vi "BarPlot.vi"(3 "Zen Analytics in":refnum<class "Zen Analytics.lvclass">, 5 "MeasuremetDisabledIndex":i32[](array[numeric]), 6 "InitializationValue-Input":T2, 7 "Plot Cluster":T1, 8 "error in (no error)":errorcluster, 9 "Graph Refference's":T3, 10 "MeasurementInitializationData.Measurement Names":string[](array[string]), 11 "Input_Data":dbl[][](array[numeric])=[[1.0, 2.0, 3.0, 4.0, 5.0, 6.0, 7.0, 8.0, 9.0, 10.0], [1.0, 2.0, 3.0, 4.0, 5.0, 6.0, 7.0, 8.0, 9.0, 10.0], [1.0, 2.0, 3.0, 4.0, 5.0, 6.0, 7.0, 8.0, 9.0, 10.0], [1.0, 2.0, 3.0, 4.0, 5.0, 6.0, 7.0, 8.0, 9.0, 10.0], [1.0, 2.0, 3.0, 4.0, 5.0, 6.0, 7.0, 8.0, 9.0, 10.0], [1.0, 2.0, 3.0, 4.0, 5.0, 6.0, 7.0, 8.0, 9.0, 10.0], [1.0, 2.0, 3.0, 4.0, 5.0, 6.0, 7.0, 8.0, 9.0, 10.0], [1.0, 2.0, 3.0, 4.0, 5.0, 6.0, 7.0, 8.0, 9.0, 10.0], [1.0, 2.0, 3.0, 4.0, 6.0, 6.0, 7.0, 8.0, 9.0, 10.0], [1.0, 2.0, 3.0, 4.0, 5.0, 6.0, 7.0, 8.0, 9.0, 10.0]]) -> (0 "error out":errorcluster, 4 "InitializationValues-Output":T2)   [LabVIEW 2019, in "Zen Analytics.lvlib" / "Zen Analytics.lvclass"]
uses:
  Zen Analytics.lvclass
  Dependency/Plot Cluster.ctl
  Dependency/GraphReff.ctl
panel:
  in  "ColorForProduction":u32[](array[colorbox])=[30476, 12845604]
  in  "ColorsForDefects":u32[](array[colorbox])=[10387, 14090395, 38587, 9764938, 14009600, 8908544, 16618491, 12294549, 16752640, 3516387, 14559999, 10192043, 7115400, 10130292, 9071204, 9961652, 2293830, 9806267, 9069692, 10138508, 9217715, 10788291, 12293525, 16512, 8388736, 8421568, 4194432, 16384, 16448, 4194304, 8405056, 5177423, 2293830]
types:
  T1 = typedef "Zen Analytics.lvlib/Zen Analytics.lvclass/Plot Cluster.ctl" = cluster{"Reduced 2D":dbl[][], "Start Index":i32, "No Of New Termnals":i32, "Top/Bottom":bool, "Values Inserted":i32, "Re-Initialised":bool, "Statistical params":string[][], "MeasurementInitializationData":cluster{"Measurement-ID":i32[], "Measurement Names":string[], "NominalValues":dbl[], "LSL":dbl[], "USL":dbl[], "LCL":dbl[], "UCL":dbl[]}, "MeasurementData":cluster{"Measurement ID":i32, "Measurement Name":string, "Nominal Values":dbl, "LSL":dbl, "USL":dbl, "LCL":dbl, "UCL":dbl}[], "ResultData2D":dbl[][], "PlotParameters":cluster{"Trend":cluster{"TrendPlotID":dbl, "PlotProperties":cluster{"FontName":string, "FontSize":dbl, "FontColor":string, "IsBold":bool, "IsItalic":bool, "PlotColor":string}}[], "Histogram":cluster{"HistogramPlotID":dbl, "PlotProperties":cluster{"FontName":string, "FontSize":dbl, "FontColor":string, "IsBold":bool, "IsItalic":bool, "PlotColor":string}}[], "BarPlot":cluster{"BarPlotID":dbl, "BarValuesID":dbl, "PlotProperties":cluster{"FontName":string, "FontSize":dbl, "IsBold":bool, "IsItalic":bool, "FontColor":string}, "Sectors":string[]}[], "PieChart":cluster{"PieChartID":dbl, "PieChartValueID":dbl, "PlotProperties":cluster{"FontName":string, "FontSize":dbl, "IsBold":bool, "IsItalic":bool, "FontColor":string}, "Sectors":string[]}[]}}
  T2 = cluster{"InitializationDefect":dbl[], "InitializationProduction":dbl[]}
  T3 = typedef "Zen Analytics.lvlib/Zen Analytics.lvclass/GraphReff.ctl" = cluster{"HistgramGraph-reff":refnum<vi>[], "BarGraph-reff":refnum<vi>[], "PieGraph-reff":refnum<vi>[], "Lable-reff":refnum<vi>[], "TrendGraph-reff":refnum<vi>[], "CpCpkTable":refnum<vi>}
  T4 = cluster{"Measurement-ID":i32[], "Measurement Names":string[], "NominalValues":dbl[], "LSL":dbl[], "USL":dbl[], "LCL":dbl[], "UCL":dbl[]}
  T5 = cluster{"BarPlotID":dbl, "BarValuesID":dbl, "PlotProperties":cluster{"FontName":string, "FontSize":dbl, "IsBold":bool, "IsItalic":bool, "FontColor":string}, "Sectors":string[]}[]
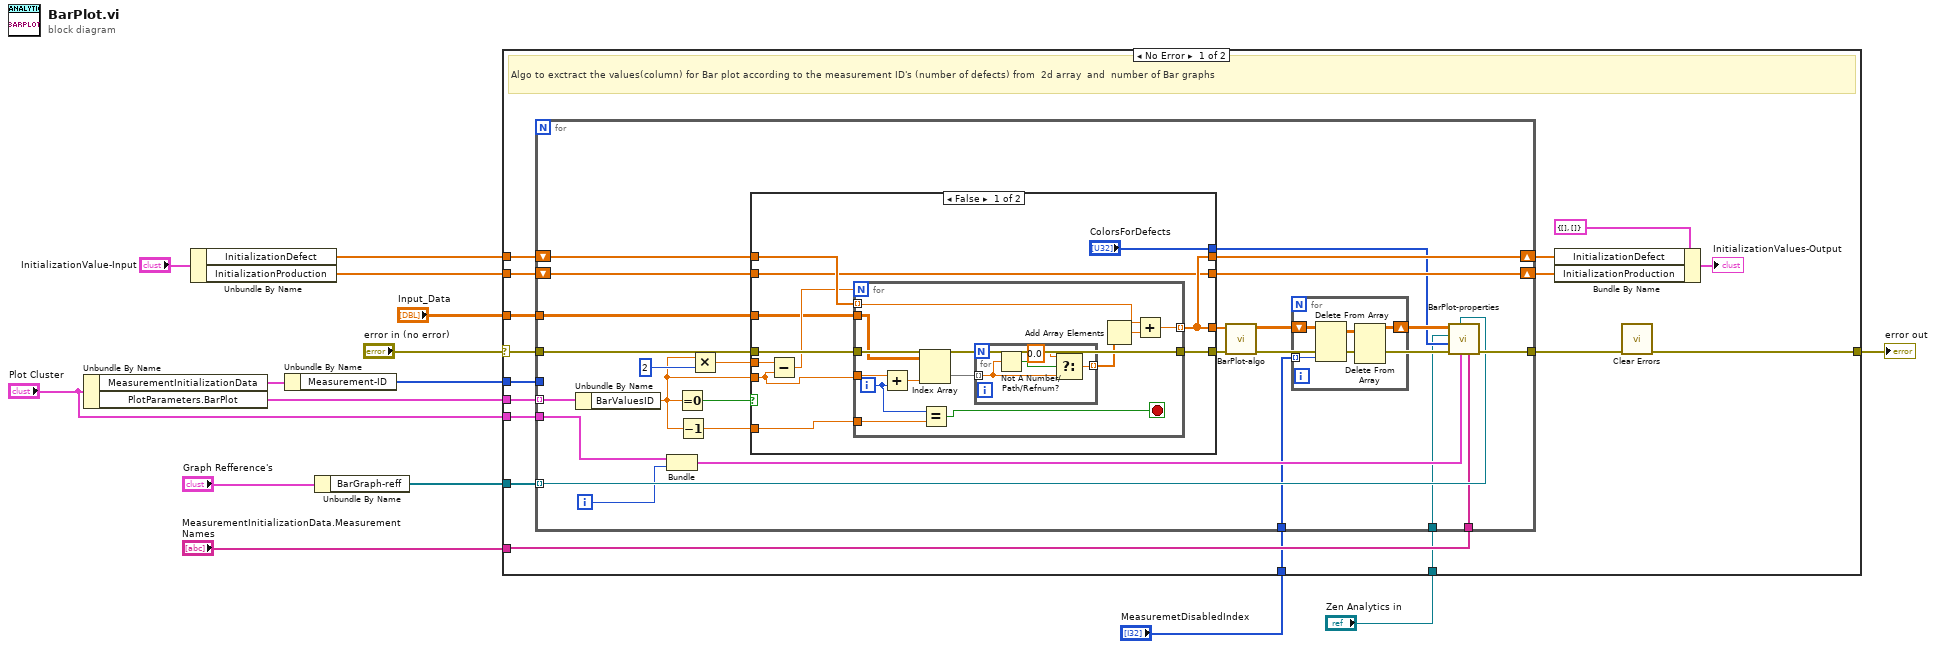
[diagram p0: block diagram]
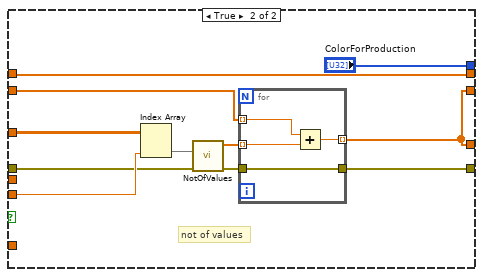
[diagram p2: hidden frame]
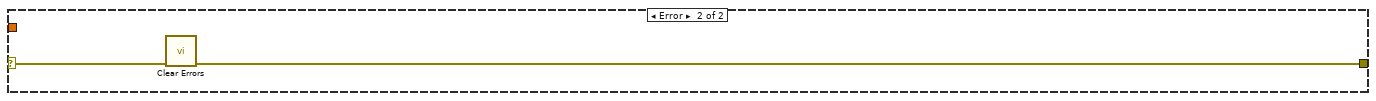
[diagram p3: hidden frame]
diagram:
  n1 = Unbundle By Name("Plot Cluster") -> ("MeasurementInitializationData"=w6:T4, "PlotParameters.BarPlot"=w9:T5)
  n2 = Unbundle By Name("InitializationValue-Input") -> ("InitializationDefect"=w2:dbl[], "InitializationProduction"=w10:dbl[])
  n3 = Unbundle By Name(w6) -> ("Measurement-ID"=w12:i32[])
  n4 = Unbundle By Name("Graph Refference's") -> ("BarGraph-reff"=w14:refnum<vi>[])
  n5 = case shown="No Error" "error in (no error)" {
    selector: "error in (no error)" -> [w29 w106]
    tunnel: [w17 w105] -> w3
    tunnel: w14 -> [w28 _]
    tunnel: w12 -> [w32 _]
    tunnel: w9 -> [w31 _]
    tunnel: "Input_Data" -> [w27 _]
    tunnel: w2 -> [w26 _]
    tunnel: w10 -> [w25 _]
    tunnel: "Plot Cluster" -> [w20 _]
    tunnel: "MeasurementInitializationData.Measurement Names" -> [w19 _]
    tunnel: "MeasuremetDisabledIndex" -> [w18 _]
    tunnel: "Zen Analytics in" -> [w16 _]
    frame No Error {
      # "Algo to exctract the values(column) for Bar plot according to the measurement ID's (number of defects) from  2d array  and  number of Bar graphs"
      n6 = for {
        tunnel: w32 -> [_]
        tunnel: w31 -> [w45] mode=indexing
        tunnel: [w58] -> w30
        tunnel: w29 -> [w57]
        tunnel: w28 -> [w56] mode=indexing
        tunnel: w27 -> [w55]
        tunnel: w20 -> [w50]
        shift-right: [w53] -> w23
        shift-left: w26 -> [w54]
        shift-right: [w51] -> w21
        shift-left: w25 -> [w52]
        tunnel: w19 -> [w46]
        tunnel: w18 -> [w42]
        tunnel: w16 -> [w33]
        i -> [w41]
        n7 = Unbundle By Name(w45) -> ("BarValuesID"=w44:dbl)
        n8 = Bundle("Plot Cluster"=w50, w41) -> (w49:cluster{"Plot Cluster":T1, i32})  [unwired: 1 in]
        n9 = Equal To 0?(x=w44) -> (x = 0?=w34:bool)
        n10 = Decrement(x=w44) -> (x-1=w48:dbl)
        n11 = Multiply(x=w44, y=2) -> (x*y=w43:dbl)
        n12 = case shown="False" w34 {
          tunnel: w55 -> [w64 w100]
          tunnel: w57 -> [w71 w91]
          tunnel: [w72 w95] -> w39
          tunnel: [w68 w94] -> w40
          tunnel: w43 -> [w73 _]
          tunnel: w44 -> [w66 w99]
          tunnel: ["ColorsForDefects" "ColorForProduction"] -> w36
          tunnel: w54 -> [w69 w97]
          tunnel: [w68 w97] -> w53
          tunnel: w52 -> [w67 w96]
          tunnel: [w67 w94] -> w51
          tunnel: w48 -> [w63 _]
          frame False {
            n13 = Subtract(x=w73, y=w66) -> (x-y=w65:dbl)
            n14 = for {
              N: w65 -> [_]
              tunnel: w66 -> [w78]
              tunnel: [w85] -> w72
              tunnel: w71 -> [w85]
              tunnel: w69 -> [w82] mode=indexing
              tunnel: [w83] -> w68 mode=indexing
              tunnel: w64 -> [w79]
              tunnel: w63 -> [w75]
              i -> [w76]
              stop <- w74 stop-if-true
              n15 = Add(x=w78, y=w76) -> (x+y=w77:dbl)
              n16 = Index Array(array=w79, index (col)=w77) -> (element=w81:dbl[])  [unwired: 1 in]
              n17 = Equal?(x=w76, y=w75) -> (x = y?=w74:bool)
              n18 = for {
                tunnel: w81 -> [w86] mode=indexing
                tunnel: [w88] -> w80 mode=indexing
                n19 = Not A Number/Path/Refnum?(number/path/refnum=w86) -> (NaN/Path/Refnum?=w87:bool)
                n20 = Select(t=0.0, s=w87, f=w86) -> (s? t:f=w88:dbl)
              }
              n21 = Add Array Elements(numeric array=w80) -> (sum=w84:dbl)
              n22 = Add(x=w82, y=w84) -> (x+y=w83:dbl)
            }
          }
          frame True {
            # "not of values"
            n23 = Index Array(array=w100, index (col)=w99) -> (element=w93:dbl[])  [unwired: 1 in]
            n24 = call "NotOfValues.vi"("error in (no error)"=w91, "Inputdata"=w93) -> ("error out"=w90:errorcluster, "Outputvalues"=w92:dbl[])  [unwired: 8 in]
            n25 = for {
              tunnel: w92 -> [w104] mode=indexing
              tunnel: [w103] -> w94 mode=indexing
              tunnel: w96 -> [w102] mode=indexing
              tunnel: w90 -> [w101]
              tunnel: [w101] -> w95
              n26 = Add(x=w102, y=w104) -> (x+y=w103:dbl)
            }
          }
        }
        n27 = call "BarPlot-algo.vi"("error in (no error)"=w39, "InputData"=w40) -> ("error out"=w38:errorcluster, "Defect Count for Top View"=w35:dbl[][])  [unwired: 8 in]
        n28 = for {
          tunnel: w42 -> [w59] mode=indexing
          shift-right: [w60] -> w37
          shift-left: w35 -> [w62]
          n29 = Delete From Array(array=w62, index (col)=w59) -> (array with subset deleted=w61:dbl[][])  [unwired: 2 in, 1 out]
          n30 = Delete From Array(array=w61, index (row)=w59) -> (array with subset deleted=w60:dbl[][])  [unwired: 2 in, 1 out]
        }
        n31 = call "BarPlot-properties.vi"("MeasurementInitializationData.Measurement Names"=w46, "Plot Cluster Index out"=w49, "Bar graph"=w56, "error in (no error)"=w38, "color"=w36, "Zen Analytics in"=w33, "BarValues"=w37) -> ("error out"=w58:errorcluster)  [unwired: 4 in]
      }
      n32 = Bundle By Name(cluster=T2 {"InitializationDefect"=[], "InitializationProduction"=[]} ("input cluster"), "InitializationDefect"=w23, "InitializationProduction"=w21) -> (→"InitializationValues-Output":T2)
      n33 = call <vilib>:"Clear Errors.vi"("error in (no error)"=w30) -> ("error out"=w17:errorcluster)  [unwired: 5 in, 1 out]
    }
    frame Error {
      n34 = call <vilib>:"Clear Errors.vi"("error in (no error)"=w106) -> ("error out"=w105:errorcluster)  [unwired: 5 in, 1 out]
    }
  }
  "error out" <- w3
